vi "build_variable_table.vi"(8 "error in (no error)":errorcluster, 11 "ExperimentVariables in":refnum<class "ExperimentVariables.lvclass">) -> (0 "error out":errorcluster, 3 "ExperimentVariables out":refnum<class "ExperimentVariables.lvclass">)   [LabVIEW 2013, in "ExperimentVariables.lvclass"]
uses:
  ExperimentVariables.lvclass
  ExperimentVariables.lvclass/ExperimentVariables.ctl
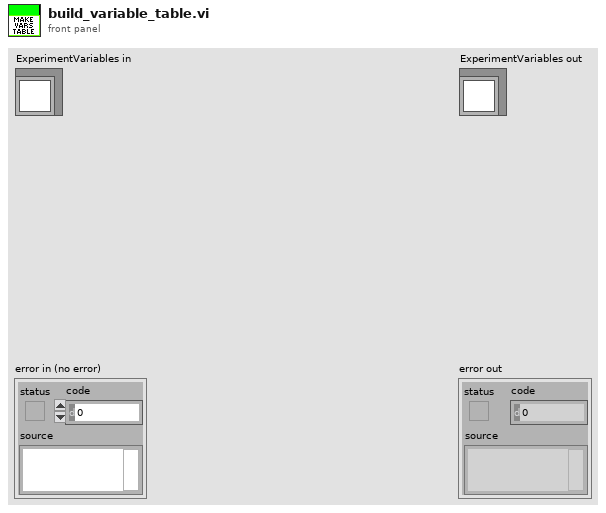
[diagram p1: front panel]
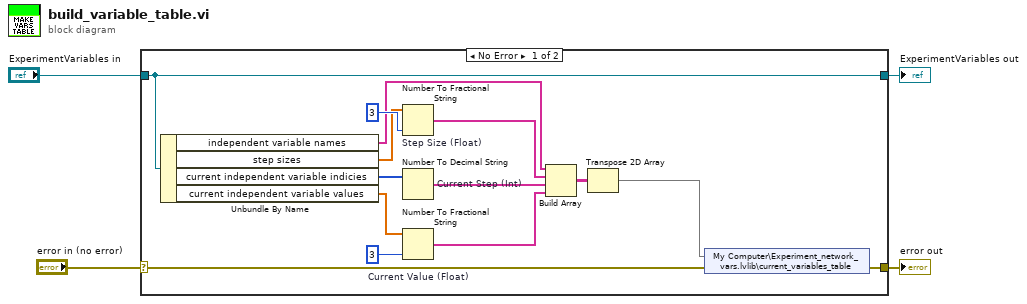
[diagram p0: block diagram]
diagram:
  n1 = case shown="No Error" "error in (no error)" {
    selector: "error in (no error)" -> [w7 w20]
    tunnel: [w5 w20] -> w3
    tunnel: [w6 w19] -> w1
    tunnel: "ExperimentVariables in" -> [w6 w19]
    frame No Error {
      n2 = Unbundle By Name(w6) -> ("independent variable names"=w12:string[], "step sizes"=w11:dbl[], "current independent variable indicies"=w10:i32[], "current independent variable values"=w9:dbl[])
      n3 = Number To Fractional String "Step Size (Float)"(number=w11, precision (6)=i16 3) -> (F-format string=w16:string[])  [unwired: 2 in]
      n4 = Number To Decimal String "Current Step (Int)"(number=w10) -> (decimal integer string=w15:string[])  [unwired: 1 in]
      n5 = Number To Fractional String "Current Value (Float)"(number=w9, precision (6)=i16 3) -> (F-format string=w14:string[])  [unwired: 2 in]
      n6 = Build Array(w12, w16, w15, w14) -> (w13:string[][])
      n7 = Transpose 2D Array(2D array=w13) -> (transposed array=w8:string[][])
      n8 = shared-variable "My Computer\\Experiment_network_vars.lvlib\\current_variables_table"(w8, error in=w7) -> (error out=w5:errorcluster)
    }
    frame Error {
    }
  }
  "error out" <- w3
  "ExperimentVariables out" <- w1
